vi "Teleop.vi"(10 "Match Info":T1={"Autonomous Elapsed Seconds"=0.0, "TeleOp Elapsed Seconds"=0.0, "Disabled Elapsed Seconds"=0.0, "Visited Autonomous"=FALSE, "Visited TeleOp"=FALSE, "Visited Disabled"=FALSE, "Autonomous Settings"={"Autonomous Style"=enum."Independent", "VI Refnum"=refnum}}, 11 "Call Context":T2) -> ()   [LabVIEW 2016]
doc: "This VI is called for each TeleOp packet received from the DS where the robot is not disabled. It is often used to read from the joysticks and update I/O or to update setpoints for timed control loops. It should complete and return within 20 milliseconds or it may miss DS packets."
uses:
  <vilib>/Rock Robotics/WPI/DriverStation/WPI_DriverStationDerivedRobotMode.ctl
  <vilib>/Rock Robotics/WPI/DriverStation/WPI_DriverStationMatch Info.ctl
  <vilib>/Rock Robotics/Network Tables/NT Read Boolean.vi
  <vilib>/Rock Robotics/Network Tables/NT Read Number.vi
  Robot Global Data.vi
  <vilib>/Rock Robotics/Network Tables/NT Write Numeric Array.vi
  <vilib>/Rock Robotics/WPI/Utilities/WPI_GetSetVariantRefNum.vi
  <vilib>/Rock Robotics/Network Tables/NT Write Boolean Array.vi
panel:
  in  "Shooter Motor Speed":dbl
  out "Sample Slider 0":dbl(slide) scale=0.0..5.0
  out "Sample Boolean 1":bool
  out "Sample Boolean 0":bool
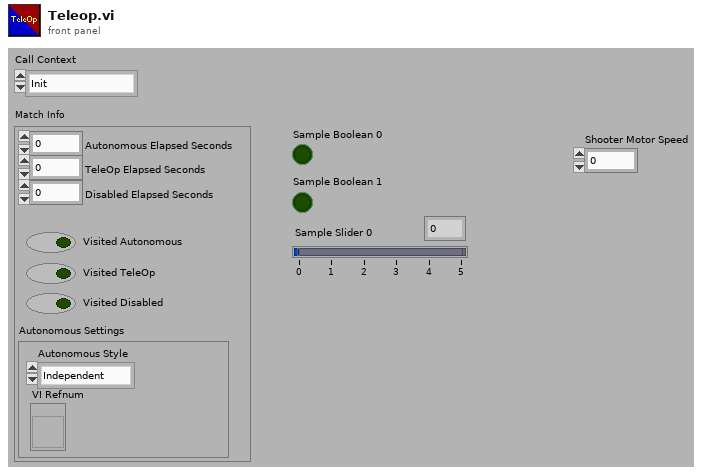
[diagram p1: front panel]
types:
  T1 = typedef "WPI_DriverStationMatch Info.ctl" = cluster{"Autonomous Elapsed Seconds":dbl, "TeleOp Elapsed Seconds":dbl, "Disabled Elapsed Seconds":dbl, "Visited Autonomous":bool, "Visited TeleOp":bool, "Visited Disabled":bool, "Autonomous Settings":cluster{"Autonomous Style":enum16{"Iterative", "Independent"}, "VI Refnum":refnum<vi>}}
  T2 = typedef "WPI_DriverStationDerivedRobotMode.ctl" = enum16{"Init", "Execute", "Stop"}
  T3 = typedef "WPI_RobotDriveDevRef.ctl" = cluster{"DevStatus":errorcluster, "Motors[]":T4[], "Square Inputs":bool, "Max Output":dbl}
  T4 = typedef "WPI_MotorControlDeviceRef.ctl" = cluster{"DeviceStatus":errorcluster, "Type":T5, "PWM":cluster{"PWM Channel":T6, "DeadBand":T7}, "CAN":cluster{"Device Number":u8, "SetOutput VI Ref":variant, "GetOutput VI Ref":variant, "Enable VI Ref":variant, "Disable VI Ref":variant, "Data":variant}, "Invert":bool}
  T5 = typedef "WPI_MotorControlType.ctl" = enum16{"PWM", "CAN"}
  T6 = typedef "FPGA_DIOPWMChannel.ctl" = enum8{"PWM 0", "PWM 1", "PWM 2", "PWM 3", "PWM 4", "PWM 5", "PWM 6", "PWM 7", "PWM 8", "PWM 9", "PWM MXP 0", "PWM MXP 1", "PWM MXP 2", "PWM MXP 3", "PWM MXP 4", "PWM MXP 5", "PWM MXP 6", "PWM MXP 7", "PWM MXP 8", "PWM MXP 9", "Invalid"}
  T7 = typedef "WPI_PWMDeadband.ctl" = cluster{"Name":string, "maxPositivePwm":i32, "minPositivePwm":i32, "centerPwm":i32, "maxNegativePwm":i32, "minNegativePwm":i32, "angularRange":u16}
  T8 = typedef "WPI_ServoDeviceRef.ctl" = cluster{"DeviceStatus":errorcluster, "PWM Channel":T6, "DeadBand":T7}
  T9 = typedef "WPI_JoystickDevRef.ctl" = cluster{"Device":T10}
  T10 = typedef "WPI_JoystickDeviceEnum.ctl" = enum16{"USB 0", "USB 1", "USB 2", "USB 3", "USB 4", "USB 5"}
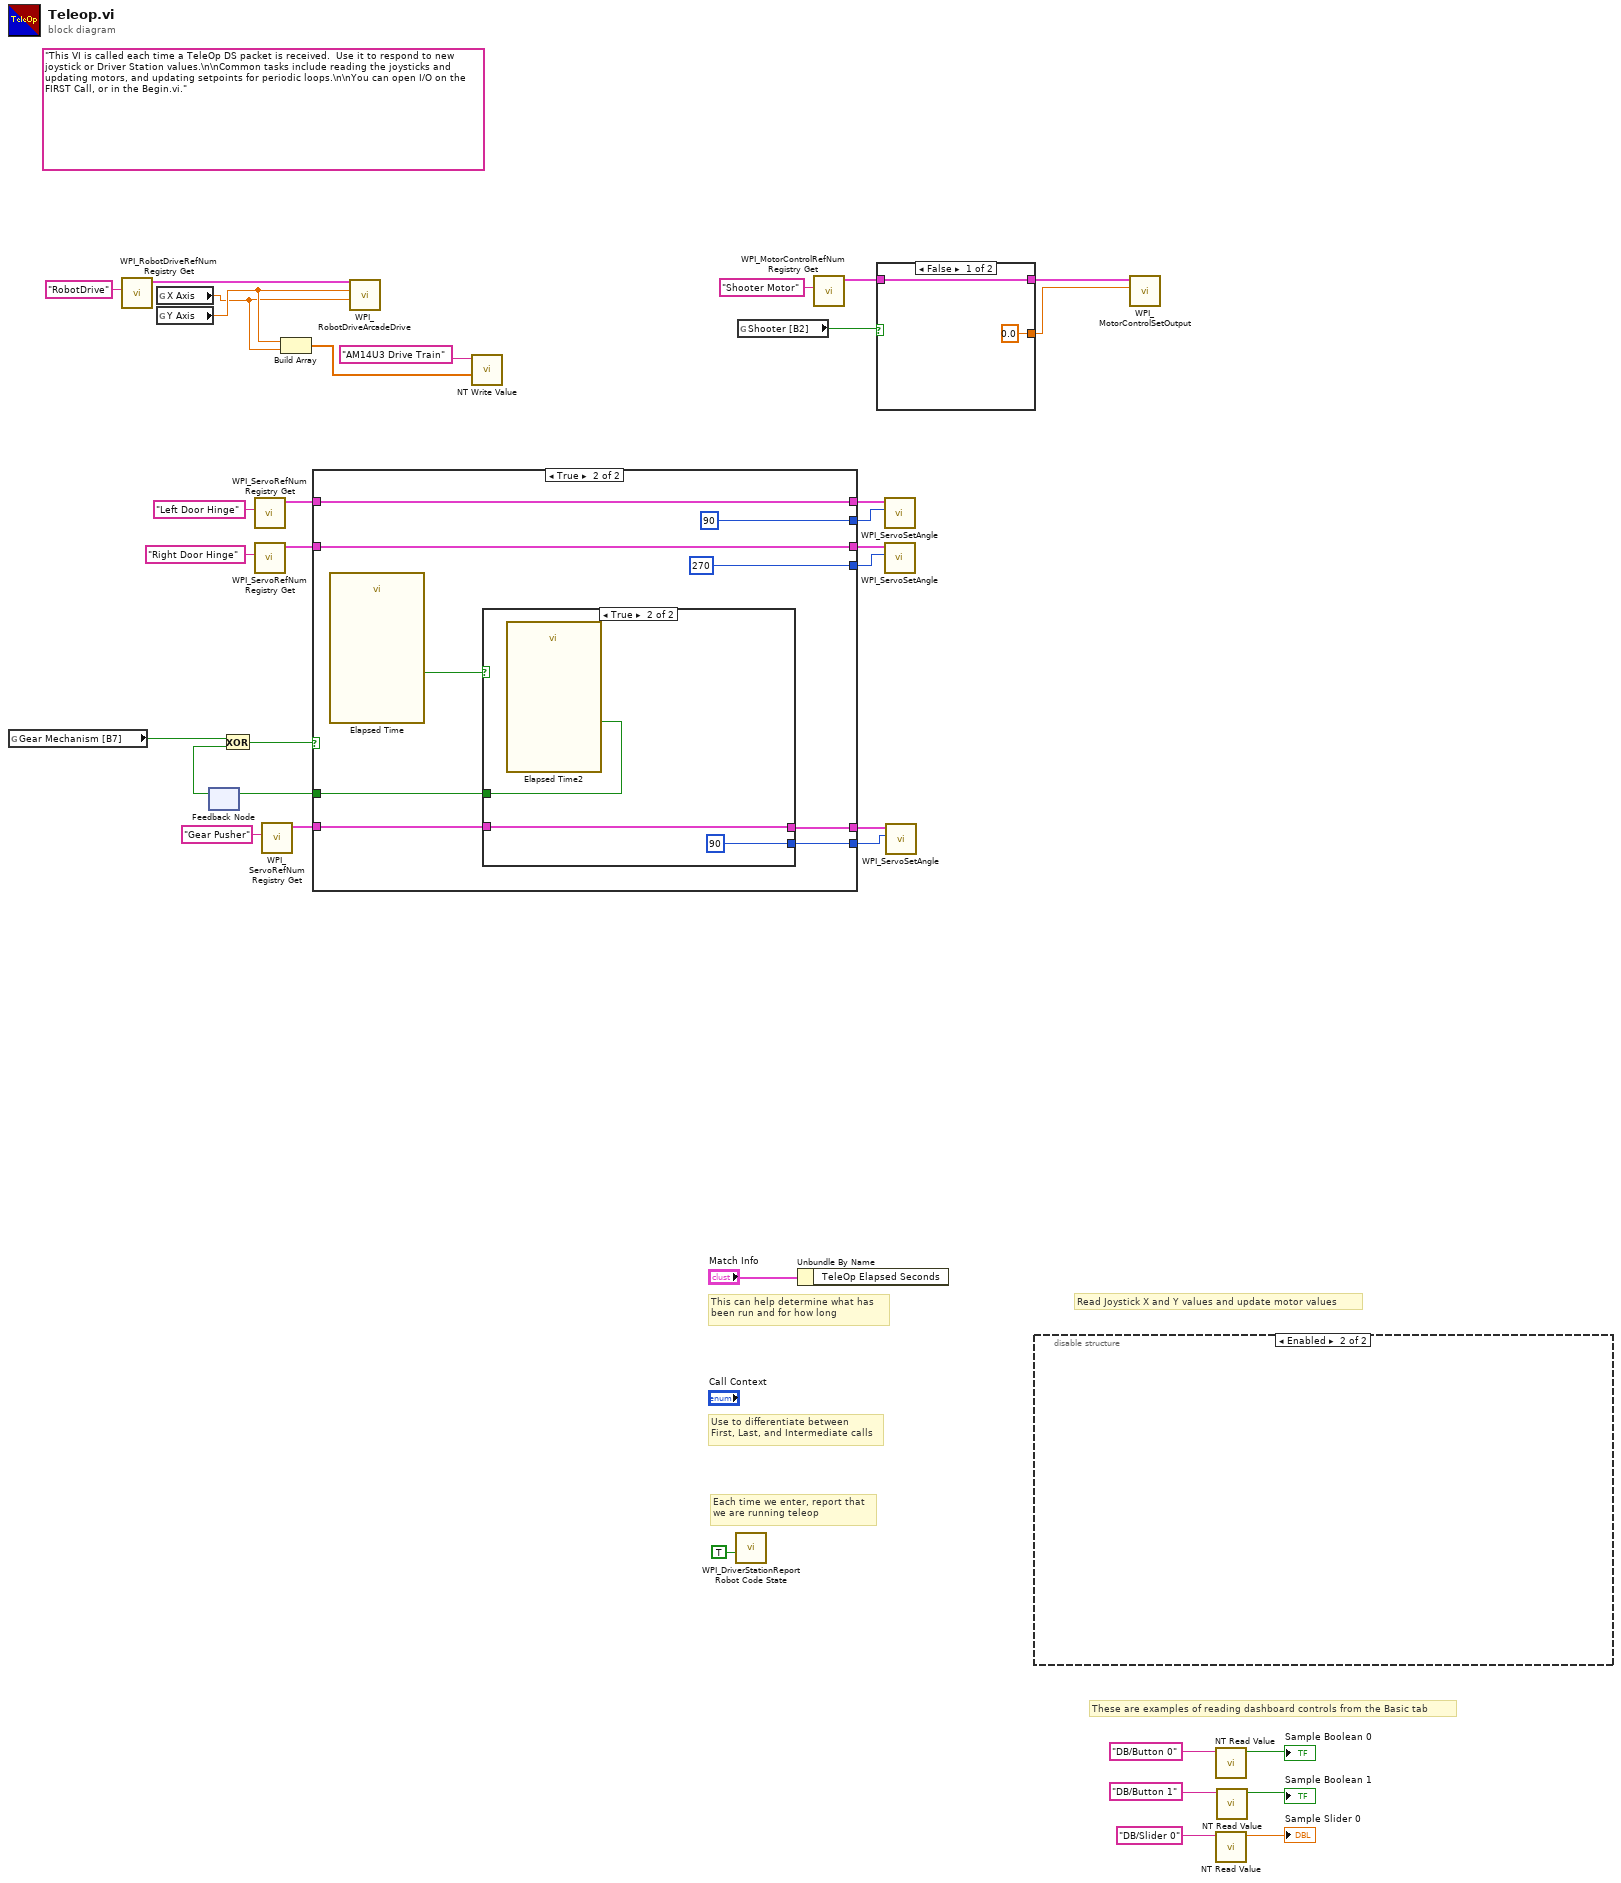
[diagram p0: block diagram]
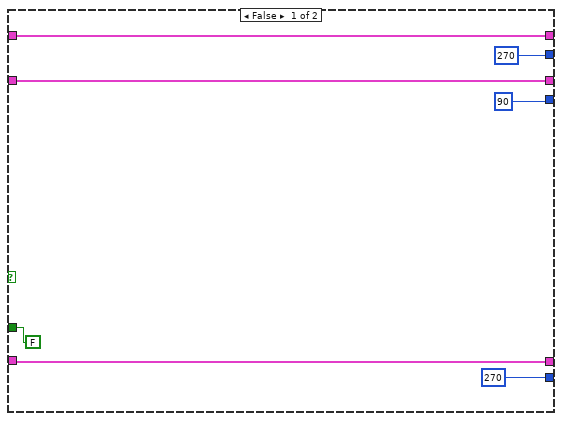
[diagram p2: hidden frame]
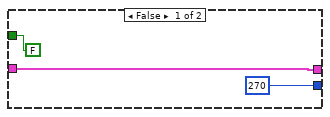
[diagram p3: hidden frame]
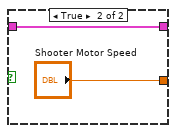
[diagram p4: hidden frame]
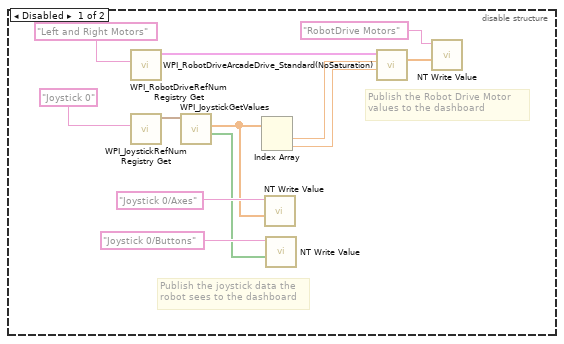
[diagram p5: hidden frame]
diagram:
  (unwired) "This VI is called each time a TeleOp DS packet is received.  Use it to respond to new joystick or Driver Station values.\n\nCommon tasks include reading the joysticks and updating motors, and updating setpoints for periodic loops.\n\nYou can open I/O on the FIRST Call, or in the Begin.vi."
  # "These are examples of reading dashboard controls from the Basic tab"
  # "Each time we enter, report that\nwe are running teleop"
  # "Use to differentiate between\nFirst, Last, and Intermediate calls"
  # "This can help determine what has\nbeen run and for how long"
  # "Read Joystick X and Y values and update motor values"
  n1 = global read "Robot Global Data.vi" "Gear Mechanism [B7]"() -> (w4:bool)
  n2 = call <vilib>:"WPI_RobotDriveRefNum Registry Get.vi"("refnum name"="RobotDrive") -> ("RobotDriveDevRef"=w26:T3)  [unwired: 9 in, 1 out]
  n3 = global read "Robot Global Data.vi" "X Axis"() -> (w17:dbl)
  n4 = global read "Robot Global Data.vi" "Y Axis"() -> (w18:dbl)
  n5 = feedback #1() -> (w1:bool)  [unwired: 1 in]
  n6 = Exclusive Or(1:w1, 2:w4) -> (0:w3:bool)
  n7 = call <vilib>:"WPI_ServoRefNum Registry Get.vi"("refnum name"="Left Door Hinge") -> ("ServoDeviceRef"=w14:T8)  [unwired: 9 in, 1 out]
  n8 = call <vilib>:"WPI_ServoRefNum Registry Get.vi"("refnum name"="Right Door Hinge") -> ("ServoDeviceRef"=w13:T8)  [unwired: 9 in, 1 out]
  n9 = call <vilib>:"WPI_ServoRefNum Registry Get.vi"("refnum name"="Gear Pusher") -> ("ServoDeviceRef"=w8:T8)  [unwired: 9 in, 1 out]
  n10 = Build Array(w18, w17) -> (w25:dbl[])
  n11 = case shown="True" w3 {
    tunnel: w14 -> [w42 w51]
    tunnel: w13 -> [w41 w50]
    tunnel: [w42 w51] -> w12
    tunnel: [w41 w50] -> w11
    tunnel: [270 90] -> w10
    tunnel: [90 270] -> w9
    tunnel: w8 -> [w38 w46]
    tunnel: [w38 w45] -> w7
    tunnel: [270 ("Angle") w44] -> w5
    tunnel: [FALSE ("Time has Elapsed") w43] -> w2
    frame False {
    }
    frame True {
      n12 = call "Elapsed Time"() -> ("Time has Elapsed"=w47:bool)  [unwired: 12 in, 7 out]
      n13 = case shown="True" w47 {
        tunnel: w46 -> [w53 w57]
        tunnel: [w53 w57] -> w45
        tunnel: [270 90] -> w44
        tunnel: [FALSE ("Time has Elapsed") w56] -> w43
        frame False {
        }
        frame True {
          n14 = call "Elapsed Time2"() -> ("Time has Elapsed"=w56:bool)  [unwired: 12 in, 7 out]
        }
      }
    }
  }
  n15 = feedback-in #1(w2) -> ()
  n16 = call-poly <vilib>:"WPI_RobotDriveArcadeDrive.vi"("Y axis value"=w17, "X axis value"=w18, "RobotDriveDevRef"=w26) -> ()  [unwired: 6 in, 3 out]
  n17 = call-poly <vilib>:"NT Write Value.vi"("Numeric Array"=w25, "Name"="AM14U3 Drive Train") -> ()  [unwired: 9 in, 1 out]
  n18 = call <vilib>:"WPI_DriverStationReport Robot Code State.vi"("TeleOp"=TRUE ("Autonomous")) -> ()  [unwired: 10 in, 1 out]
  n19 = global read "Robot Global Data.vi" "Shooter [B2]"() -> (w22:bool)
  n20 = Unbundle By Name("Match Info") -> ()  [unwired: 1 out]
  n21 = call <vilib>:"WPI_MotorControlRefNum Registry Get.vi"("refnum name"="Shooter Motor") -> ("MotorControlDevRef"=w21:T4)  [unwired: 9 in, 1 out]
  n22 = case shown="False" w22 {
    tunnel: w21 -> [w58 w61]
    tunnel: [w58 w61] -> w20
    tunnel: [0.0 ("Shooter Motor Speed") "Shooter Motor Speed"] -> w19
    frame False {
    }
    frame True {
    }
  }
  n23 = call <vilib>:"WPI_ServoSetAngle.vi"("Angle"=w10, "ServoDeviceRef"=w12) -> ()  [unwired: 8 in, 2 out]
  n24 = call <vilib>:"WPI_ServoSetAngle.vi"("Angle"=w9, "ServoDeviceRef"=w11) -> ()  [unwired: 8 in, 2 out]
  n25 = call <vilib>:"WPI_ServoSetAngle.vi"("Angle"=w5, "ServoDeviceRef"=w7) -> ()  [unwired: 8 in, 2 out]
  n26 = disable-structure shown="Enabled" {
    frame Disabled {
      # "Publish the Robot Drive Motor\nvalues to the dashboard"
      # "Publish the joystick data the\nrobot sees to the dashboard"
      n27 = call <vilib>:"WPI_RobotDriveRefNum Registry Get.vi"("refnum name"="Left and Right Motors") -> ("RobotDriveDevRef"=w72:T3)  [unwired: 1 in, 9 out]
      n28 = call <vilib>:"WPI_JoystickRefNum Registry Get.vi"("refnum name"="Joystick 0") -> ("JoystickDevRef"=w69:T9)  [unwired: 1 in, 9 out]
      n29 = call <vilib>:"WPI_JoystickGetValues.vi"("JoystickDevRef"=w69) -> ("Buttons"=w64:bool[], "Axes"=w65:dbl[])  [unwired: 6 in, 3 out]
      n30 = Index Array(array=w65) -> (element #1=w71:dbl, element #2=w68:dbl)  [unwired: 2 in]
      n31 = call-poly <vilib>:"NT Write Value.vi"("Numeric Array"=w65, "Name"="Joystick 0/Axes") -> ()  [unwired: 9 in, 1 out]
      n32 = call-poly <vilib>:"NT Write Value.vi"("Boolean Array"=w64, "Name"="Joystick 0/Buttons") -> ()  [unwired: 9 in, 1 out]
      n33 = call <vilib>:"WPI_RobotDriveArcadeDrive_Standard(NoSaturation).vi"("Y axis value"=w68, "X axis value"=w71, "RobotDriveDevRef"=w72) -> ("Motor Values"=w63:dbl[])  [unwired: 1 in, 7 out]
      n34 = call-poly <vilib>:"NT Write Value.vi"("Numeric Array"=w63, "Name"="RobotDrive Motors") -> ()  [unwired: 9 in, 1 out]
    }
    frame Enabled {
    }
  }
  n35 = call <vilib>:"WPI_MotorControlSetOutput.vi"("Output"=w19, "MotorControlDevRef"=w20) -> ()  [unwired: 7 in, 3 out]
  n36 = call-poly <vilib>:"NT Read Value.vi"("Name"="DB/Button 0" ("refnum name")) -> ("Boolean"=→"Sample Boolean 0":bool)  [unwired: 9 in, 1 out]
  n37 = call-poly <vilib>:"NT Read Value.vi"("Name"="DB/Slider 0" ("refnum name")) -> ("Numeric"=→"Sample Slider 0":dbl)  [unwired: 9 in, 1 out]
  n38 = call-poly <vilib>:"NT Read Value.vi"("Name"="DB/Button 1" ("refnum name")) -> ("Boolean"=→"Sample Boolean 1":bool)  [unwired: 9 in, 1 out]
